vi "Sort 2D Array.vi"(9 "Sort by Datatype Array":enum16{"String", "Number", "Date-Time"}[](array[ring]), 10 "Sort by Cols":i32[](array[numeric])=[1, 2], 11 "Input Array":string[][](array[string])=[["ID03172011132910", "D11014", "B5", "1", "Crystal CdTe", "CZT EXP009", "0.0143", "2", "3/17/2011 1:29:10 PM", "dtester", "0.1", "25", "Custom - Uses option tab setting", "1155", "161.6", "3/17/2011 1:24:56 PM", "5/25/2010 1:00:00 PM", "", "ID03172011132910", "0.000018331135", "0.329199646", "-0.000019162902", "0.290582012", "12248.694", "23122.247", "0.000001833114", "0.179016841", "0.000010239894", "0", "0.992889686", "8.68126209E-46", "4.422637E-12", "4451299", "-131.960127", "61928.868", "", "", "", "", ""], ["ID03172011133056", "D11014", "B5", "2", "Crystal CdTe", "CZT EXP009", "0.0143", "1", "3/17/2011 1:30:56 PM", "dtester", "0.1", "25", "Custom - Uses option tab setting", "1155", "161.6", "3/17/2011 1:24:56 PM", "5/25/2010 1:00:00 PM", "", "ID03172011133056", "0.000019774033", "0.343694416", "-0.000019403825", "0.29650732", "11605.468", "24816.221", "0.000001977403", "0.188833978", "0.00001047165", "3222.311", "0.992305147", "4.10762544E-46", "4.64417E-12", "5095988", "-116.319344", "80376.492", "", "", "", "", ""], ["ID03172011134450", "D11016", "E4", "1", "Crystal CdTe", "CZT EXP009", "0.0143", "2", "3/17/2011 1:44:50 PM", "dtester", "0.1", "25", "Custom - Uses option tab setting", "0", "161.6", "3/17/2011 1:24:56 PM", "5/25/2010 1:00:00 PM", "", "ID03172011134450", "0", "0.066337846", "-0.000001549743", "0", "24000.955", "355279.503", "0", "0", "0", "0", "0.932694566", "4.712838E-48", "1.521848E-12", "100000000000000", "-1301.062", "361382.131", "", "", "", "", ""], ["ID03172011134552", "D11016", "E4", "2", "Crystal CdTe", "CZT EXP009", "0.0143", "1", "3/17/2011 1:45:52 PM", "dtester", "0.1", "25", "Custom - Uses option tab setting", "0", "161.6", "3/17/2011 1:24:56 PM", "5/25/2010 1:00:00 PM", "", "ID03172011134552", "0.000001609791", "0.18902661", "-0.000004209879", "0.202291173", "55653.293", "29563.168", "0.0000001609791", "0.093729707", "0.000001717482", "0", "0.836775618", "3.606545E-48", "0.000000003769194", "100000000000000", "-504.246188", "546040.796", "", "", "", "", ""], ["ID03172011134725", "D11017", "A3", "1", "Crystal CdTe", "CZT EXP009", "0.0143", "1", "3/17/2011 1:47:25 PM", "dtester", "0.1", "25", "Custom - Uses option tab setting", "0", "161.6", "3/17/2011 1:24:56 PM", "5/25/2010 1:00:00 PM", "", "ID03172011134725", "0.000007862703", "0.300634425", "-0.000009351238", "0.279681693", "25122.784", "37448.672", "0.00000078627026", "0.161786792", "0.000004859916", "0", "0.998501747", "1.881718E-48", "3.03841765E-10", "7111744", "-173.547592", "554111.9", "", "", "", "", ""], ["ID03172011134847", "D11017", "A3", "3", "Crystal CdTe", "CZT EXP009", "0.0143", "1", "3/17/2011 1:48:47 PM", "dtester", "0.1", "25", "Custom - Uses option tab setting", "0", "161.6", "3/17/2011 1:24:56 PM", "5/25/2010 1:00:00 PM", "", "ID03172011134847", "0.000007726846", "0.299639907", "-0.000009106517", "0.283171979", "25227.847", "39025.402", "0.000000772684597", "0.161170617", "0.000004794203", "29301660", "0.996689983", "9.30590943E-49", "8.7875222E-11", "7981629", "-169.139745", "676093.501", "", "", "", "", ""], ["ID03172011135004", "D11016", "E2", "1", "Crystal CdTe", "CZT EXP009", "0.0143", "1", "3/17/2011 1:50:04 PM", "dtester", "0.1", "25", "Custom - Uses option tab setting", "0", "161.6", "3/17/2011 1:24:56 PM", "5/25/2010 1:00:00 PM", "", "ID03172011135004", "0.000008887575", "0.314422094", "-0.000011008741", "0.256763078", "24162.056", "38566.512", "0.000000888757533", "0.135568669", "0.000006555774", "372634.151", "0.99877204", "2.5938593E-47", "1.00830354E-10", "6315776", "-188.727106", "224030.183", "", "", "", "", ""], ["ID03172011135102", "D11016", "E2", "2", "Crystal CdTe", "CZT EXP009", "0.0143", "1", "3/17/2011 1:51:02 PM", "dtester", "0.1", "25", "Custom - Uses option tab setting", "0", "161.6", "3/17/2011 1:24:56 PM", "5/25/2010 1:00:00 PM", "", "ID03172011135102", "0.000008220737", "0.299774635", "-0.000008826217", "0.310700021", "23973.842", "26397.011", "0.000000822073702", "0.180441307", "0.000004555906", "0", "0.998383932", "2.0025352E-47", "1.04854738E-10", "6274781", "-214.846448", "244423.023", "", "", "", "", ""], ["ID03172011135230", "D11017", "C1", "1", "Crystal CdTe", "CZT EXP009", "0.0143", "1", "3/17/2011 1:52:30 PM", "dtester", "0.1", "25", "Custom - Uses option tab setting", "0", "161.6", "3/17/2011 1:24:56 PM", "5/25/2010 1:00:00 PM", "", "ID03172011135230", "0.000009002015", "0.322095736", "-0.000010017559", "0.278992685", "25552.404", "38853.628", "0.000000900201474", "0.172166433", "0.00000522867", "16809035", "0.998577656", "5.83859492E-49", "3.0578151E-10", "7303523", "-156.257879", "798891.399", "", "", "", "", ""], ["ID03172011135446", "D11014", "A2", "1", "Crystal CdTe", "CZT EXP009", "0.0143", "1", "3/17/2011 1:54:46 PM", "dtester", "0.1", "25", "Custom - Uses option tab setting", "0", "161.6", "3/17/2011 1:24:56 PM", "5/25/2010 1:00:00 PM", "retry", "ID03172011135446", "0.000008121558", "0.318938896", "-0.000008607329", "0.295844468", "25228.235", "29753.235", "0.000000812155756", "0.158334247", "0.000005129375", "0", "0.996400609", "2.016331E-48", "3.99575382E-10", "9290112", "-74.919625", "546763.331", "", "", "", "", ""], ["ID03172011135542", "D11014", "A2", "2", "Crystal CdTe", "CZT EXP009", "0.0143", "1", "3/17/2011 1:55:42 PM", "dtester", "0.1", "25", "Custom - Uses option tab setting", "0", "162", "3/17/2011 1:24:56 PM", "5/25/2010 1:00:00 PM", "retry", "ID03172011135542", "0.000010769773", "0.316532242", "-0.000010678727", "0.31861711", "18332.836", "32777.717", "0.000001076977", "0.185023821", "0.000005820749", "0", "0.994541054", "3.879299E-48", "9.0565763E-11", "8933675", "-113.837654", "437235.26", "", "", "", "", ""], ["ID03172011135702", "D11016", "C3", "1", "Crystal CdTe", "CZT EXP009", "0.0143", "1", "3/17/2011 1:57:02 PM", "dtester", "0.1", "25", "Custom - Uses option tab setting", "0", "161.6", "3/17/2011 1:24:56 PM", "5/25/2010 1:00:00 PM", "retry", "ID03172011135702", "0.000005099675", "0.235096132", "-0.000007926189", "0.27367339", "25734.358", "34044.701", "0.000000509967465", "0.123146343", "0.00000414115", "4091317000", "0.989780648", "6.5732986E-50", "0.00000012792339", "6862941", "-258.957329", "1691082", "", "", "", "", ""], ["ID03172011135800", "D11016", "C3", "2", "Crystal CdTe", "CZT EXP009", "0.0143", "1", "3/17/2011 1:58:00 PM", "dtester", "0.1", "25", "Custom - Uses option tab setting", "0", "161.6", "3/17/2011 1:24:56 PM", "5/25/2010 1:00:00 PM", "retry", "ID03172011135800", "0.000006572242", "0.277556032", "-0.00000897193", "0.263922873", "36049.094", "36545.224", "0.000000657224249", "0.14400509", "0.000004563896", "4327975000000", "0.969663856", "1.11030837E-52", "3.012567E-14", "205688100", "-168.692902", "9146911", "", "", "", "", ""]]) -> (3 "Output Array":string[][](array[string])=[["ID03172011135446", "D11014", "A2", "1", "Crystal CdTe", "CZT EXP009", "0.0143", "1", "3/17/2011 1:54:46 PM", "dtester", "0.1", "25", "Custom - Uses option tab setting", "0", "161.6", "3/17/2011 1:24:56 PM", "5/25/2010 1:00:00 PM", "retry", "ID03172011135446", "0.000008121558", "0.318938896", "-0.000008607329", "0.295844468", "25228.235", "29753.235", "0.000000812155756", "0.158334247", "0.000005129375", "0", "0.996400609", "2.016331E-48", "3.99575382E-10", "9290112", "-74.919625", "546763.331", "", "", "", "", "", "", "", "", "", "", "", "", "", "", ""], ["ID03172011135542", "D11014", "A2", "2", "Crystal CdTe", "CZT EXP009", "0.0143", "1", "3/17/2011 1:55:42 PM", "dtester", "0.1", "25", "Custom - Uses option tab setting", "0", "162", "3/17/2011 1:24:56 PM", "5/25/2010 1:00:00 PM", "retry", "ID03172011135542", "0.000010769773", "0.316532242", "-0.000010678727", "0.31861711", "18332.836", "32777.717", "0.000001076977", "0.185023821", "0.000005820749", "0", "0.994541054", "3.879299E-48", "9.0565763E-11", "8933675", "-113.837654", "437235.26", "", "", "", "", "", "", "", "", "", "", "", "", "", "", ""], ["ID03172011132910", "D11014", "B5", "1", "Crystal CdTe", "CZT EXP009", "0.0143", "2", "3/17/2011 1:29:10 PM", "dtester", "0.1", "25", "Custom - Uses option tab setting", "1155", "161.6", "3/17/2011 1:24:56 PM", "5/25/2010 1:00:00 PM", "", "ID03172011132910", "0.000018331135", "0.329199646", "-0.000019162902", "0.290582012", "12248.694", "23122.247", "0.000001833114", "0.179016841", "0.000010239894", "0", "0.992889686", "8.68126209E-46", "4.422637E-12", "4451299", "-131.960127", "61928.868", "", "", "", "", "", "", "", "", "", "", "", "", "", "", ""], ["ID03172011133056", "D11014", "B5", "2", "Crystal CdTe", "CZT EXP009", "0.0143", "1", "3/17/2011 1:30:56 PM", "dtester", "0.1", "25", "Custom - Uses option tab setting", "1155", "161.6", "3/17/2011 1:24:56 PM", "5/25/2010 1:00:00 PM", "", "ID03172011133056", "0.000019774033", "0.343694416", "-0.000019403825", "0.29650732", "11605.468", "24816.221", "0.000001977403", "0.188833978", "0.00001047165", "3222.311", "0.992305147", "4.10762544E-46", "4.64417E-12", "5095988", "-116.319344", "80376.492", "", "", "", "", "", "", "", "", "", "", "", "", "", "", ""], ["ID03172011135702", "D11016", "C3", "1", "Crystal CdTe", "CZT EXP009", "0.0143", "1", "3/17/2011 1:57:02 PM", "dtester", "0.1", "25", "Custom - Uses option tab setting", "0", "161.6", "3/17/2011 1:24:56 PM", "5/25/2010 1:00:00 PM", "retry", "ID03172011135702", "0.000005099675", "0.235096132", "-0.000007926189", "0.27367339", "25734.358", "34044.701", "0.000000509967465", "0.123146343", "0.00000414115", "4091317000", "0.989780648", "6.5732986E-50", "0.00000012792339", "6862941", "-258.957329", "1691082", "", "", "", "", "", "", "", "", "", "", "", "", "", "", ""], ["ID03172011135800", "D11016", "C3", "2", "Crystal CdTe", "CZT EXP009", "0.0143", "1", "3/17/2011 1:58:00 PM", "dtester", "0.1", "25", "Custom - Uses option tab setting", "0", "161.6", "3/17/2011 1:24:56 PM", "5/25/2010 1:00:00 PM", "retry", "ID03172011135800", "0.000006572242", "0.277556032", "-0.00000897193", "0.263922873", "36049.094", "36545.224", "0.000000657224249", "0.14400509", "0.000004563896", "4327975000000", "0.969663856", "1.11030837E-52", "3.012567E-14", "205688100", "-168.692902", "9146911", "", "", "", "", "", "", "", "", "", "", "", "", "", "", ""], ["ID03172011135004", "D11016", "E2", "1", "Crystal CdTe", "CZT EXP009", "0.0143", "1", "3/17/2011 1:50:04 PM", "dtester", "0.1", "25", "Custom - Uses option tab setting", "0", "161.6", "3/17/2011 1:24:56 PM", "5/25/2010 1:00:00 PM", "", "ID03172011135004", "0.000008887575", "0.314422094", "-0.000011008741", "0.256763078", "24162.056", "38566.512", "0.000000888757533", "0.135568669", "0.000006555774", "372634.151", "0.99877204", "2.5938593E-47", "1.00830354E-10", "6315776", "-188.727106", "224030.183", "", "", "", "", "", "", "", "", "", "", "", "", "", "", ""], ["ID03172011135102", "D11016", "E2", "2", "Crystal CdTe", "CZT EXP009", "0.0143", "1", "3/17/2011 1:51:02 PM", "dtester", "0.1", "25", "Custom - Uses option tab setting", "0", "161.6", "3/17/2011 1:24:56 PM", "5/25/2010 1:00:00 PM", "", "ID03172011135102", "0.000008220737", "0.299774635", "-0.000008826217", "0.310700021", "23973.842", "26397.011", "0.000000822073702", "0.180441307", "0.000004555906", "0", "0.998383932", "2.0025352E-47", "1.04854738E-10", "6274781", "-214.846448", "244423.023", "", "", "", "", "", "", "", "", "", "", "", "", "", "", ""], ["ID03172011134450", "D11016", "E4", "1", "Crystal CdTe", "CZT EXP009", "0.0143", "2", "3/17/2011 1:44:50 PM", "dtester", "0.1", "25", "Custom - Uses option tab setting", "0", "161.6", "3/17/2011 1:24:56 PM", "5/25/2010 1:00:00 PM", "", "ID03172011134450", "0", "0.066337846", "-0.000001549743", "0", "24000.955", "355279.503", "0", "0", "0", "0", "0.932694566", "4.712838E-48", "1.521848E-12", "100000000000000", "-1301.062", "361382.131", "", "", "", "", "", "", "", "", "", "", "", "", "", "", ""], ["ID03172011134552", "D11016", "E4", "2", "Crystal CdTe", "CZT EXP009", "0.0143", "1", "3/17/2011 1:45:52 PM", "dtester", "0.1", "25", "Custom - Uses option tab setting", "0", "161.6", "3/17/2011 1:24:56 PM", "5/25/2010 1:00:00 PM", "", "ID03172011134552", "0.000001609791", "0.18902661", "-0.000004209879", "0.202291173", "55653.293", "29563.168", "0.0000001609791", "0.093729707", "0.000001717482", "0", "0.836775618", "3.606545E-48", "0.000000003769194", "100000000000000", "-504.246188", "546040.796", "", "", "", "", "", "", "", "", "", "", "", "", "", "", ""], ["ID03172011134725", "D11017", "A3", "1", "Crystal CdTe", "CZT EXP009", "0.0143", "1", "3/17/2011 1:47:25 PM", "dtester", "0.1", "25", "Custom - Uses option tab setting", "0", "161.6", "3/17/2011 1:24:56 PM", "5/25/2010 1:00:00 PM", "", "ID03172011134725", "0.000007862703", "0.300634425", "-0.000009351238", "0.279681693", "25122.784", "37448.672", "0.00000078627026", "0.161786792", "0.000004859916", "0", "0.998501747", "1.881718E-48", "3.03841765E-10", "7111744", "-173.547592", "554111.9", "", "", "", "", "", "", "", "", "", "", "", "", "", "", ""], ["ID03172011134847", "D11017", "A3", "3", "Crystal CdTe", "CZT EXP009", "0.0143", "1", "3/17/2011 1:48:47 PM", "dtester", "0.1", "25", "Custom - Uses option tab setting", "0", "161.6", "3/17/2011 1:24:56 PM", "5/25/2010 1:00:00 PM", "", "ID03172011134847", "0.000007726846", "0.299639907", "-0.000009106517", "0.283171979", "25227.847", "39025.402", "0.000000772684597", "0.161170617", "0.000004794203", "29301660", "0.996689983", "9.30590943E-49", "8.7875222E-11", "7981629", "-169.139745", "676093.501", "", "", "", "", "", "", "", "", "", "", "", "", "", "", ""], ["ID03172011135230", "D11017", "C1", "1", "Crystal CdTe", "CZT EXP009", "0.0143", "1", "3/17/2011 1:52:30 PM", "dtester", "0.1", "25", "Custom - Uses option tab setting", "0", "161.6", "3/17/2011 1:24:56 PM", "5/25/2010 1:00:00 PM", "", "ID03172011135230", "0.000009002015", "0.322095736", "-0.000010017559", "0.278992685", "25552.404", "38853.628", "0.000000900201474", "0.172166433", "0.00000522867", "16809035", "0.998577656", "5.83859492E-49", "3.0578151E-10", "7303523", "-156.257879", "798891.399", "", "", "", "", "", "", "", "", "", "", "", "", "", "", ""]])   [LabVIEW 2010]
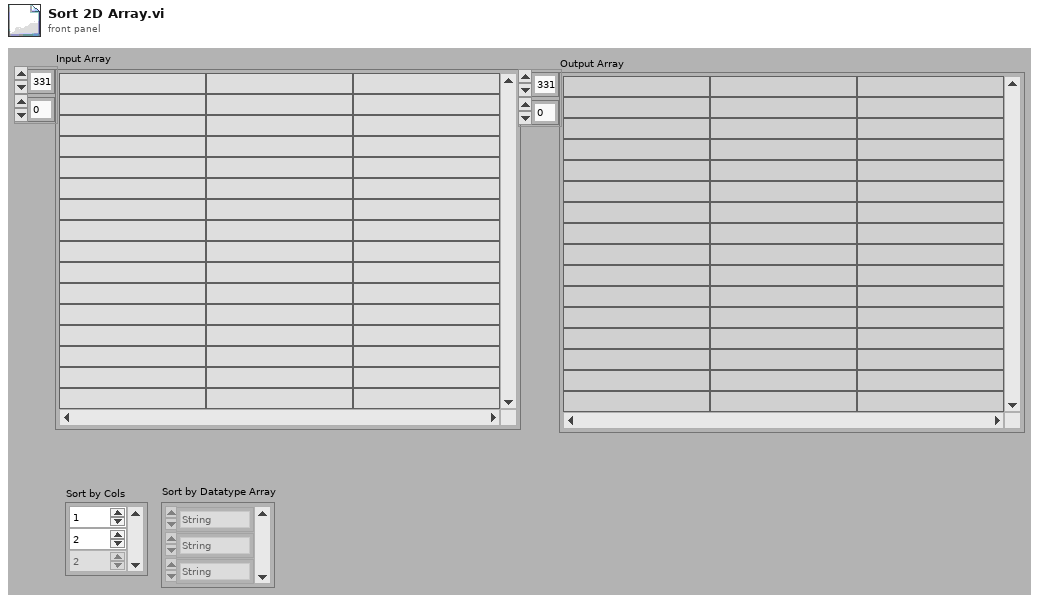
[diagram p1: front panel]
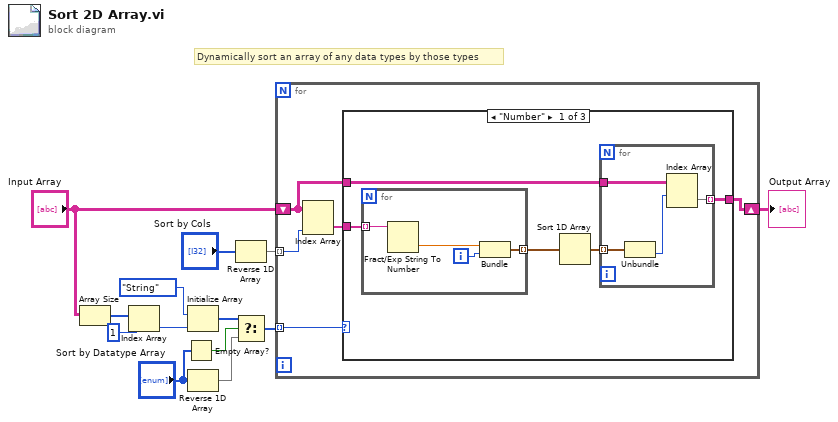
[diagram p0: block diagram]
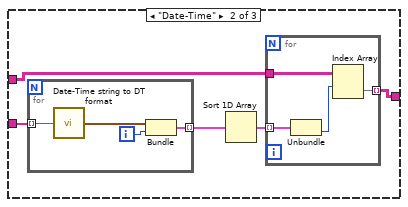
[diagram p2: hidden frame]
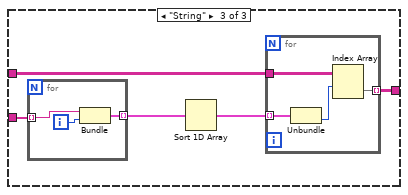
[diagram p3: hidden frame]
diagram:
  # "Dynamically sort an array of any data types by those types"
  n1 = Array Size(array="Input Array") -> (size(s)=w5:i32[])
  n2 = Index Array(array=w5, index=1) -> (element=w3:i32)
  n3 = Empty Array?(array="Sort by Datatype Array") -> (empty?=w10:bool)
  n4 = Initialize Array(enum16{"String", "Number", "Date-Time"}."String" ("Sort Type"), w3) -> (w2:enum16{"String", "Number", "Date-Time"}[])
  n5 = Reverse 1D Array(array="Sort by Datatype Array") -> (reversed array=w7:enum16{"String", "Number", "Date-Time"}[])
  n6 = Reverse 1D Array(array="Sort by Cols") -> (reversed array=w12:i32[])
  n7 = Select(t=w2, s=w10, f=w7) -> (s? t:f=w9:enum16{"String", "Number", "Date-Time"}[])
  n8 = for {
    tunnel: w12 -> [w18] mode=indexing
    tunnel: w9 -> [w16] mode=indexing
    shift-right: [w15] -> w11
    shift-left: "Input Array" -> [w14]
    n9 = Index Array(array=w14, index (col)=w18) -> (element=w17:string[])  [unwired: 1 in]
    n10 = case shown="\"Number\"" w16 {
      tunnel: w17 -> [w22 w35 w49]
      tunnel: [w21 w34 w48] -> w15
      tunnel: w14 -> [w19 w32 w46]
      frame "Number" {
        n11 = for {
          tunnel: w22 -> [w26] mode=indexing
          tunnel: [w24] -> w20 mode=indexing
          i -> [w27]
          n12 = Fract/Exp String To Number(string=w26) -> (number=w25:dbl)  [unwired: 3 in, 1 out]
          n13 = Bundle(w25, w27) -> (w24:cluster{dbl, i32})  [unwired: 1 in]
        }
        n14 = Sort 1D Array(array=w20) -> (sorted array=w23:cluster{dbl, i32}[])
        n15 = for {
          tunnel: w23 -> [w31] mode=indexing
          tunnel: w19 -> [w30]
          tunnel: [w29] -> w21 mode=indexing
          n16 = Unbundle(w31) -> (w28:i32)  [unwired: 1 out]
          n17 = Index Array(array=w30, index (row)=w28) -> (element=w29:string[])  [unwired: 1 in]
        }
      }
      frame "Date-Time" {
        n18 = for {
          tunnel: w35 -> [w38] mode=indexing
          tunnel: [w39] -> w33 mode=indexing
          i -> [w40]
          n19 = call "Date-Time string to DT format.vi"("date/time string"=w38) -> ("Resulting Time Stamp"=w37:timestamp)
          n20 = Bundle("Resulting Time Stamp"=w37, w40) -> (w39:cluster{"Resulting Time Stamp":timestamp, i32})  [unwired: 1 in]
        }
        n21 = Sort 1D Array(array=w33) -> (sorted array=w36:cluster{"Resulting Time Stamp":timestamp, i32}[])
        n22 = for {
          tunnel: w36 -> [w44] mode=indexing
          tunnel: w32 -> [w43]
          tunnel: [w42] -> w34 mode=indexing
          n23 = Unbundle(w44) -> (w41:i32)  [unwired: 1 out]
          n24 = Index Array(array=w43, index (row)=w41) -> (element=w42:string[])  [unwired: 1 in]
        }
      }
      frame "String" {
        n25 = for {
          tunnel: w49 -> [w50] mode=indexing
          tunnel: [w51] -> w47 mode=indexing
          i -> [w52]
          n26 = Bundle("String"=w50, w52) -> (w51:cluster{"String":string, i32})  [unwired: 1 in]
        }
        n27 = Sort 1D Array(array=w47) -> (sorted array=w45:cluster{"String":string, i32}[])
        n28 = for {
          tunnel: w45 -> [w56] mode=indexing
          tunnel: w46 -> [w55]
          tunnel: [w54] -> w48 mode=indexing
          n29 = Unbundle(w56) -> (w53:i32)  [unwired: 1 out]
          n30 = Index Array(array=w55, index (row)=w53) -> (element=w54:string[])  [unwired: 1 in]
        }
      }
    }
  }
  "Output Array" <- w11
